vi "RESTful Check for Invalid ASCII Characters.vi"(8 "error in (no error)":errorcluster, 11 "Parameter Name":string) -> (0 "error out":errorcluster, 3 "dup Parameter Name":string)   [LabVIEW 2020]
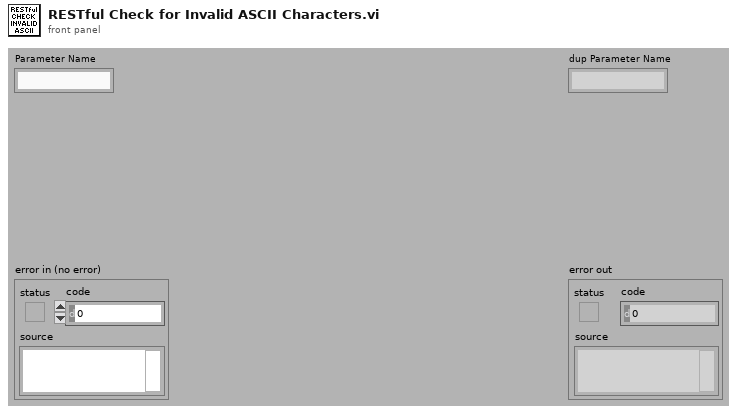
[diagram p1: front panel]
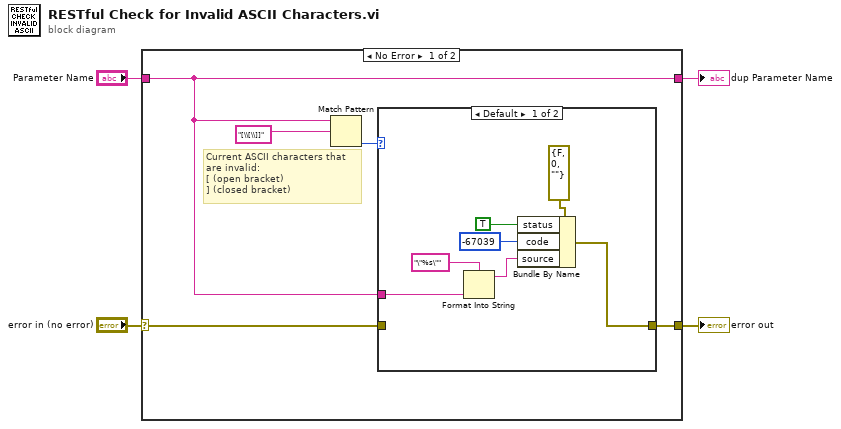
[diagram p0: block diagram]
diagram:
  n1 = case shown="No Error" "error in (no error)" {
    selector: "error in (no error)" -> [w8 w19]
    tunnel: [w6 w19] -> w3
    tunnel: "Parameter Name" -> [w5 w18]
    tunnel: [w5 w18] -> w2
    frame No Error {
      # "Current ASCII characters that are invalid:\n[ (open bracket)\n] (closed bracket)"
      n2 = Match Pattern(string=w5, regular expression="[\\[\\]]") -> (offset past match=w7:i32)  [unwired: 1 in, 3 out]
      n3 = case shown="Default" w7 {
        tunnel: w8 -> [_ w17]
        tunnel: [w12 w17] -> w6
        tunnel: w5 -> [w11 _]
        frame Default {
          n4 = Format Into String(format string="\"%s\"", w11) -> (resulting string=w13:string)  [unwired: 2 in, 1 out]
          n5 = Bundle By Name(cluster=errorcluster {"status"=FALSE, "code"=0, "source"=""} ("error in (no error)"), "status"=TRUE, "code"=-67039 ("error code (0)"), "source"=w13) -> (w12:errorcluster)
        }
        frame -1 {
        }
      }
    }
    frame Error {
    }
  }
  "error out" <- w3
  "dup Parameter Name" <- w2
